vi "Hahn & RF pi vs no pi contrast Pulse Sequence Generator.vi"(0 "N Loop":i32=10000, 1 "Rabi Frequency":dbl, 2 "RF Pulse":dbl, 3 "Tau":dbl, 5 "AOM Pulse length":dbl=2.5e-06, 7 "AOM Rest time":dbl=1e-06, 9 "Signal Delay":dbl=6e-07, 11 "APD signal width":dbl=5e-07, 12 "MW Delay":dbl, 13 "Pulse offset":dbl) -> (4 "Pulse Sequence":T1(array[cluster]))   [LabVIEW 2012]
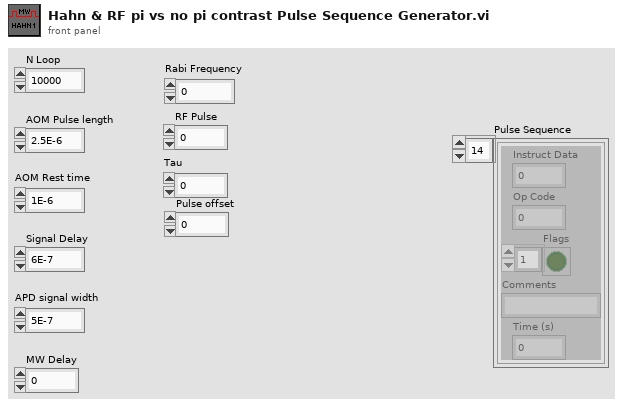
[diagram p1: front panel]
types:
  T1 = cluster{"Instruct Data":i32, "Op Code":i32, "Flags":bool[], "Comments":string, "Time (s)":dbl}[]
  T2 = cluster{"Instruct Data":i32, "Op Code":i32, "Flags":bool[], "Comments":string, "Time (s)":dbl}
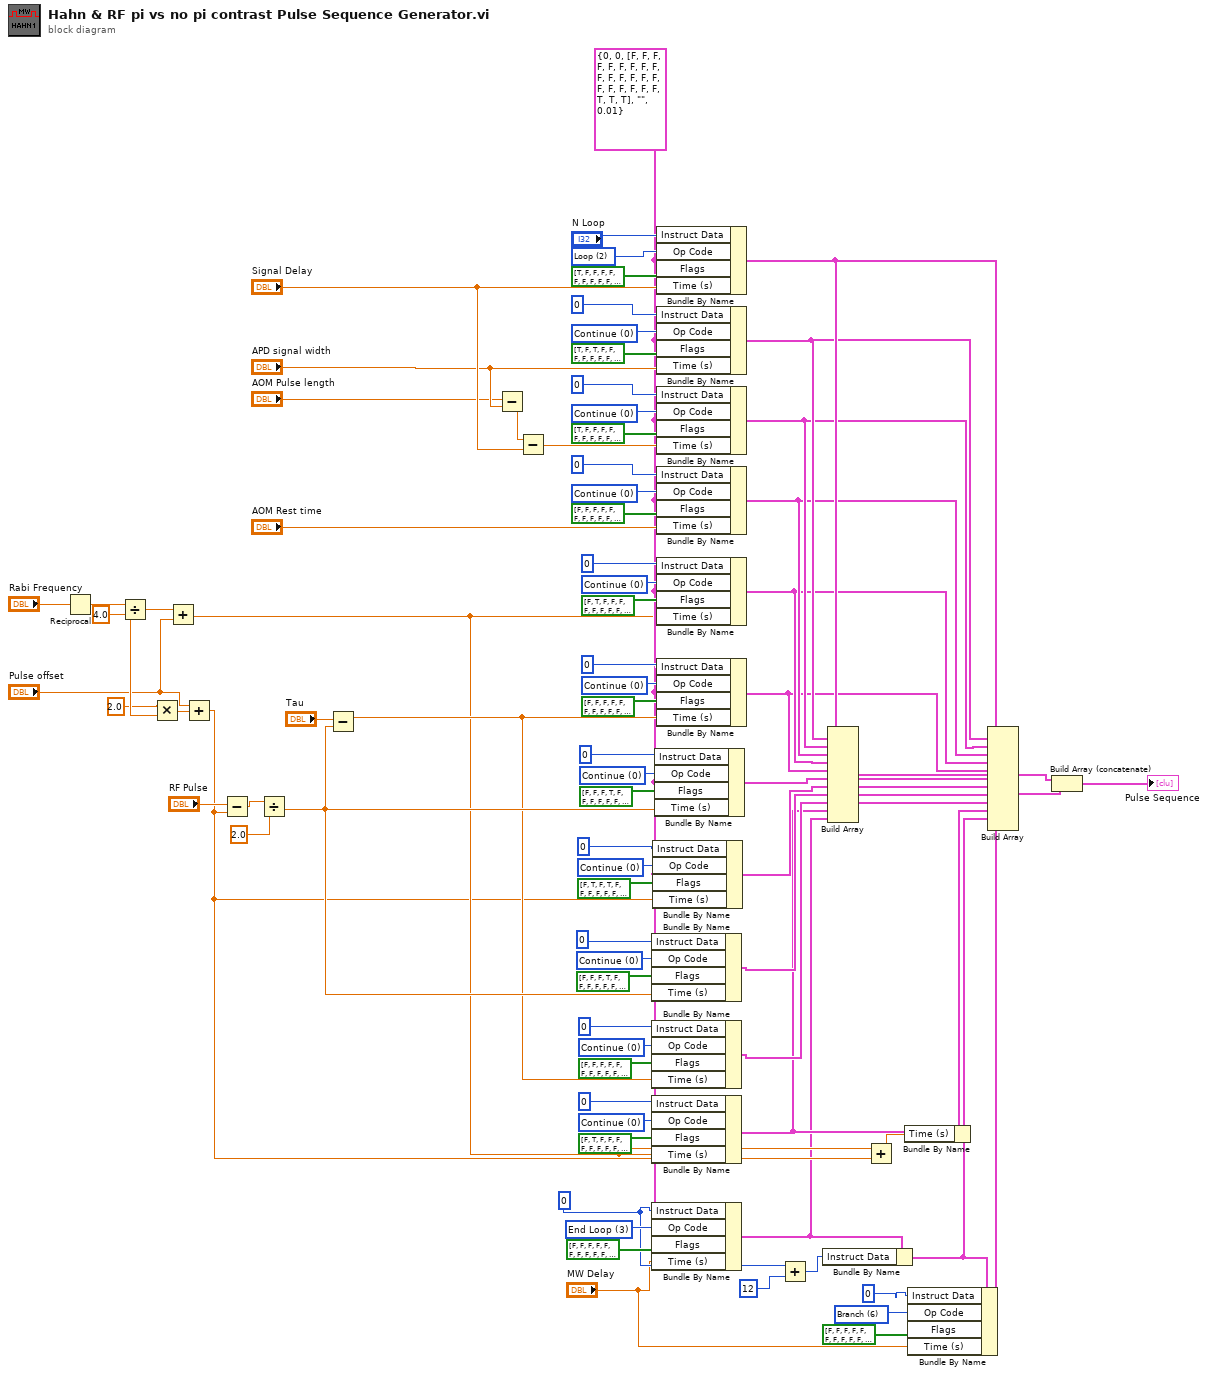
[diagram p0: block diagram]
diagram:
  w5 = 6 items=["Continue", "Stop", "Loop", "End Loop", "JSR", "RTS", "Branch", "Long Delay", "Wait"] ("Op Code")
  w22 = 0 items=["Continue", "Stop", "Loop", "End Loop", "JSR", "RTS", "Branch", "Long Delay", "Wait"] ("Op Code")
  w25 = 0 items=["Continue", "Stop", "Loop", "End Loop", "JSR", "RTS", "Branch", "Long Delay", "Wait"] ("Op Code")
  w34 = 0 items=["Continue", "Stop", "Loop", "End Loop", "JSR", "RTS", "Branch", "Long Delay", "Wait"] ("Op Code")
  w37 = 0 items=["Continue", "Stop", "Loop", "End Loop", "JSR", "RTS", "Branch", "Long Delay", "Wait"] ("Op Code")
  w41 = 0 items=["Continue", "Stop", "Loop", "End Loop", "JSR", "RTS", "Branch", "Long Delay", "Wait"] ("Op Code")
  w44 = 0 items=["Continue", "Stop", "Loop", "End Loop", "JSR", "RTS", "Branch", "Long Delay", "Wait"] ("Op Code")
  w47 = 0 items=["Continue", "Stop", "Loop", "End Loop", "JSR", "RTS", "Branch", "Long Delay", "Wait"] ("Op Code")
  w63 = 3 items=["Continue", "Stop", "Loop", "End Loop", "JSR", "RTS", "Branch", "Long Delay", "Wait"] ("Op Code")
  w18 = 0 ("y")
  w68 = 0 items=["Continue", "Stop", "Loop", "End Loop", "JSR", "RTS", "Branch", "Long Delay", "Wait"] ("Op Code")
  w72 = 0 items=["Continue", "Stop", "Loop", "End Loop", "JSR", "RTS", "Branch", "Long Delay", "Wait"] ("Op Code")
  w75 = 0 items=["Continue", "Stop", "Loop", "End Loop", "JSR", "RTS", "Branch", "Long Delay", "Wait"] ("Op Code")
  w77 = 2 items=["Continue", "Stop", "Loop", "End Loop", "JSR", "RTS", "Branch", "Long Delay", "Wait"] ("Op Code")
  w19 = T2 {"Instruct Data"=0, "Op Code"=0, "Flags"=[FALSE, FALSE, FALSE, FALSE, FALSE, FALSE, FALSE, FALSE, FALSE, FALSE, FALSE, FALSE, FALSE, FALSE, FALSE, FALSE, FALSE, FALSE, FALSE, FALSE, FALSE, TRUE, TRUE, TRUE], "Comments"="", "Time (s)"=0.01} ("PB Inst 2")
  n1 = Reciprocal(x="Rabi Frequency") -> (1/x=w52:dbl)
  n2 = Divide(x=w52, y=4.0) -> (x/y=w51:dbl)
  n3 = Multiply(x=2.0, y=w51) -> (x*y=w39:dbl)
  n4 = Add(x=w51, y="Pulse offset") -> (x+y=w10:dbl)
  n5 = Add(x="Pulse offset", y=w39) -> (x+y=w9:dbl)
  n6 = Subtract(x="RF Pulse", y=w9) -> (x-y=w30:dbl)
  n7 = Divide(x=w30, y=2.0) -> (x/y=w27:dbl)
  n8 = Subtract(x="Tau", y=w27) -> (x-y=w20:dbl)
  n9 = Subtract(x="AOM Pulse length", y="APD signal width") -> (x-y=w70:dbl)
  n10 = Subtract(x=w70, y="Signal Delay") -> (x-y=w66:dbl)
  n11 = Bundle By Name(cluster=w19, "Instruct Data"=0, "Op Code"=w34, "Flags"=bool[] [FALSE, FALSE, FALSE, TRUE, FALSE, FALSE, FALSE, FALSE, FALSE, FALSE, FALSE, FALSE, FALSE, FALSE, FALSE, FALSE, FALSE, FALSE, FALSE, FALSE, FALSE, TRUE, TRUE, TRUE], "Time (s)"=w27) -> (w13:T2)
  n12 = Bundle By Name(cluster=w19, "Instruct Data"=0, "Op Code"=w25, "Flags"=bool[] [FALSE, FALSE, FALSE, FALSE, FALSE, FALSE, FALSE, FALSE, FALSE, FALSE, FALSE, FALSE, FALSE, FALSE, FALSE, FALSE, FALSE, FALSE, FALSE, FALSE, FALSE, TRUE, TRUE, TRUE], "Time (s)"=w20) -> (w12:T2)
  n13 = Bundle By Name(cluster=w19, "Instruct Data"=0, "Op Code"=w22, "Flags"=bool[] [FALSE, TRUE, FALSE, FALSE, FALSE, FALSE, FALSE, FALSE, FALSE, FALSE, FALSE, FALSE, FALSE, FALSE, FALSE, FALSE, FALSE, FALSE, FALSE, FALSE, FALSE, TRUE, TRUE, TRUE], "Time (s)"=w10) -> (w11:T2)
  n14 = Bundle By Name(cluster=w19, "Instruct Data"=w18, "Op Code"=w63, "Flags"=bool[] [FALSE, FALSE, FALSE, FALSE, FALSE, FALSE, FALSE, FALSE, FALSE, FALSE, FALSE, FALSE, FALSE, FALSE, FALSE, FALSE, FALSE, FALSE, FALSE, FALSE, FALSE, TRUE, TRUE, TRUE], "Time (s)"="MW Delay") -> (w8:T2)
  n15 = Bundle By Name(cluster=w19, "Instruct Data"=0, "Op Code"=w37, "Flags"=bool[] [FALSE, TRUE, FALSE, TRUE, FALSE, FALSE, FALSE, FALSE, FALSE, FALSE, FALSE, FALSE, FALSE, FALSE, FALSE, FALSE, FALSE, FALSE, FALSE, FALSE, FALSE, TRUE, TRUE, TRUE], "Time (s)"=w9) -> (w14:T2)
  n16 = Bundle By Name(cluster=w19, "Instruct Data"=0, "Op Code"=w41, "Flags"=bool[] [FALSE, FALSE, FALSE, TRUE, FALSE, FALSE, FALSE, FALSE, FALSE, FALSE, FALSE, FALSE, FALSE, FALSE, FALSE, FALSE, FALSE, FALSE, FALSE, FALSE, FALSE, TRUE, TRUE, TRUE], "Time (s)"=w27) -> (w15:T2)
  n17 = Bundle By Name(cluster=w19, "Instruct Data"="N Loop", "Op Code"=w77, "Flags"=bool[] [TRUE, FALSE, FALSE, FALSE, FALSE, FALSE, FALSE, FALSE, FALSE, FALSE, FALSE, FALSE, FALSE, FALSE, FALSE, FALSE, FALSE, FALSE, FALSE, FALSE, FALSE, TRUE, TRUE, TRUE], "Time (s)"="Signal Delay") -> (w62:T2)
  n18 = Bundle By Name(cluster=w19, "Instruct Data"=0, "Op Code"=w75, "Flags"=bool[] [TRUE, FALSE, TRUE, FALSE, FALSE, FALSE, FALSE, FALSE, FALSE, FALSE, FALSE, FALSE, FALSE, FALSE, FALSE, FALSE, FALSE, FALSE, FALSE, FALSE, FALSE, TRUE, TRUE, TRUE], "Time (s)"="APD signal width") -> (w61:T2)
  n19 = Bundle By Name(cluster=w19, "Instruct Data"=0, "Op Code"=w72, "Flags"=bool[] [TRUE, FALSE, FALSE, FALSE, FALSE, FALSE, FALSE, FALSE, FALSE, FALSE, FALSE, FALSE, FALSE, FALSE, FALSE, FALSE, FALSE, FALSE, FALSE, FALSE, FALSE, TRUE, TRUE, TRUE], "Time (s)"=w66) -> (w60:T2)
  n20 = Bundle By Name(cluster=w19, "Instruct Data"=0, "Op Code"=w68, "Flags"=bool[] [FALSE, FALSE, FALSE, FALSE, FALSE, FALSE, FALSE, FALSE, FALSE, FALSE, FALSE, FALSE, FALSE, FALSE, FALSE, FALSE, FALSE, FALSE, FALSE, FALSE, FALSE, TRUE, TRUE, TRUE], "Time (s)"="AOM Rest time") -> (w59:T2)
  n21 = Bundle By Name(cluster=w19, "Instruct Data"=0, "Op Code"=w47, "Flags"=bool[] [FALSE, TRUE, FALSE, FALSE, FALSE, FALSE, FALSE, FALSE, FALSE, FALSE, FALSE, FALSE, FALSE, FALSE, FALSE, FALSE, FALSE, FALSE, FALSE, FALSE, FALSE, TRUE, TRUE, TRUE], "Time (s)"=w10) -> (w17:T2)
  n22 = Bundle By Name(cluster=w19, "Instruct Data"=0, "Op Code"=w44, "Flags"=bool[] [FALSE, FALSE, FALSE, FALSE, FALSE, FALSE, FALSE, FALSE, FALSE, FALSE, FALSE, FALSE, FALSE, FALSE, FALSE, FALSE, FALSE, FALSE, FALSE, FALSE, FALSE, TRUE, TRUE, TRUE], "Time (s)"=w20) -> (w16:T2)
  n23 = Add(x=w18, y=12) -> (x+y=w56:i32)
  n24 = Bundle By Name(cluster=w8, "Instruct Data"=w56) -> (w2:T2)
  n25 = Build Array(w62, w61, w60, w59, w17, w16, w15, w14, w13, w12, w11, w8) -> (w55:T1)
  n26 = Add(x=w10, y=w9) -> (x+y=w58:dbl)
  n27 = Bundle By Name(cluster=w11, "Time (s)"=w58) -> (w7:T2)
  n28 = Bundle By Name(cluster=w2, "Instruct Data"=0 ("y"), "Op Code"=w5, "Flags"=bool[] [FALSE, FALSE, FALSE, FALSE, FALSE, FALSE, FALSE, FALSE, FALSE, FALSE, FALSE, FALSE, FALSE, FALSE, FALSE, FALSE, FALSE, FALSE, FALSE, FALSE, FALSE, TRUE, TRUE, TRUE], "Time (s)"="MW Delay") -> (w3:T2)
  n29 = Build Array(w62, w61, w60, w59, w17, w16, w15, w14, w13, w12, w7, w2, w3) -> (w54:T1)
  n30 = Build Array (concatenate)(w55, w54) -> (→"Pulse Sequence":T1)
